vi "MB Open Connection.vi"(11 "Test Object in":T1) -> (0 "error out":errorcluster, 3 "Test Object out":T1)   [LabVIEW 2021]
uses:
  TypeDefs/Tester Object.ctl
  <vilib>/NI/Modbus Library/API/Master/Modbus Master.lvclass
  TypeDefs/UIControlReferences.ctl
  <vilib>/Utility/config.llb/Read Key (String).vi
  <vilib>/Utility/config.llb/Read Key (U32).vi
  <vilib>/NI/Modbus Library/API/Wrapper/Create Serial Master.vi
  <vilib>/NI/Modbus Library/API/Wrapper/Create TCP Master.vi
  <vilib>/regexp/Match Regular Expression.xnode
  <vilib>/NI/Modbus Library/API/Wrapper/API Main.lvlib
  <vilib>/Utility/config.llb/NI_LVConfig.lvlib
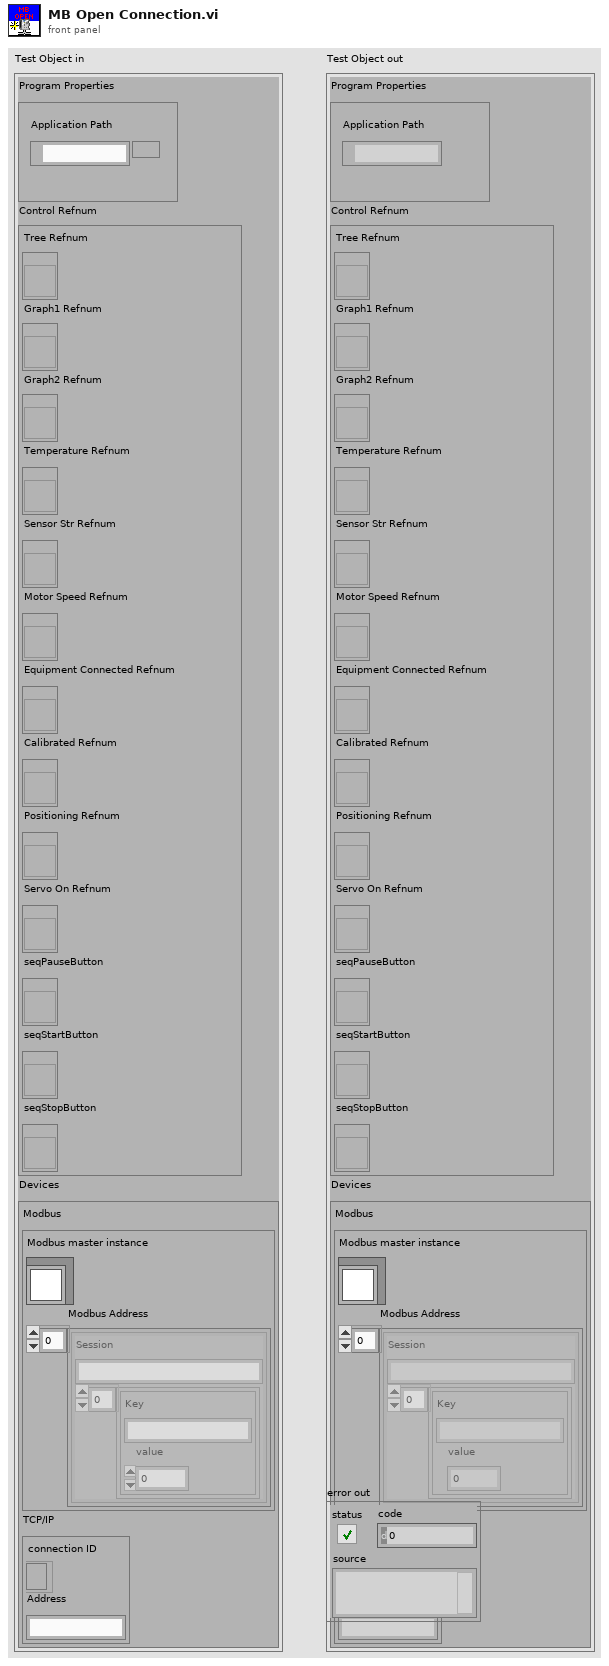
[diagram p1: front panel]
types:
  T1 = typedef "Tester Object.ctl" = cluster{"Program Properties":cluster{"Application Path":path}, "Control Refnum":T2, "Devices":cluster{"Modbus":cluster{"Modbus master instance":refnum<class "Modbus Master.lvclass">, "Modbus Address":cluster{"Session":string, cluster{"Key":string, "value":u32}[]}[]}, "TCP/IP":cluster{"connection ID":refnum<k5>, "Address":string}}}
  T2 = typedef "UIControlReferences.ctl" = cluster{"Tree Refnum ":refnum<vi>, "Graph1 Refnum":refnum<vi>, "Graph2 Refnum":refnum<vi>, "Temperature Refnum":refnum<vi>, "Sensor Str Refnum":refnum<vi>, "Motor Speed Refnum":refnum<vi>, "Equipment Connected Refnum":refnum<vi>, "Calibrated Refnum":refnum<vi>, "Positioning Refnum":refnum<vi>, "Servo On Refnum":refnum<vi>, "seqPauseButton":refnum<vi>, "seqStartButton":refnum<vi>, "seqStopButton":refnum<vi>}
  T3 = typedef "NI_LVConfig.lvlib/Config Data RefNum.ctl" = refnum<k1>
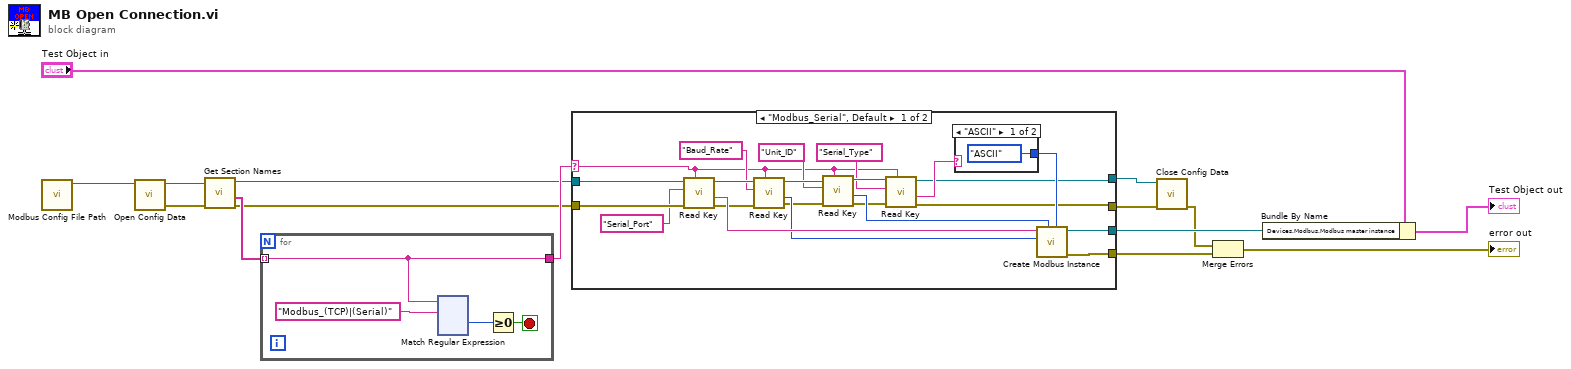
[diagram p0: block diagram]
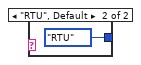
[diagram p2: hidden frame]
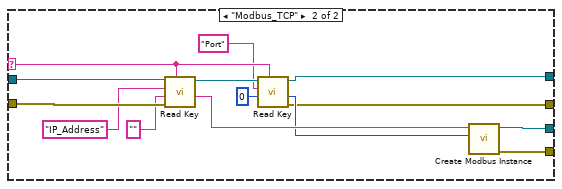
[diagram p3: hidden frame]
diagram:
  n1 = call "Modbus Config File Path.vi"() -> ("appended path out"=w15:path)  [unwired: 11 in]
  n2 = call <vilib>:"Open Config Data.vi"("configuration file path"=w15) -> ("error out"=w13:errorcluster, "refnum"=w14:T3)  [unwired: 8 in, 1 out]
  n3 = call <vilib>:"Get Section Names.vi"("error in (no error)"=w13, "refnum"=w14) -> ("error out"=w9:errorcluster, "section names"=w12:string[], "refnum out"=w10:T3)  [unwired: 7 in]
  n4 = for {
    tunnel: w12 -> [w16] mode=indexing
    tunnel: [w16] -> w11
    stop <- w18 stop-if-true
    n5 = xnode "Match Regular Expression"("input string"=w16, "regular expression"="Modbus_(TCP)|(Serial)") -> ("offset past match"=w17:i32)  [unwired: 4 in, 4 out]
    n6 = Greater Or Equal To 0?(x=w17) -> (x >= 0?=w18:bool)
  }
  n7 = case shown="\"Modbus_Serial\", Default" w11 {
    selector: w11 -> [w141 w167]
    tunnel: w10 -> [w158 w172]
    tunnel: w9 -> [w157 w171]
    tunnel: [w156 w173] -> w6
    tunnel: [w155 w174] -> w5
    tunnel: [w138 w162] -> w4
    tunnel: [w137 w161] -> w3
    frame "Modbus_Serial", Default {
      n8 = call-poly <vilib>:"Read Key.vi"("section"=w141, "error in (no error)"=w157, "key"="Serial_Port", "refnum"=w158) -> ("error out"=w151:errorcluster, "value"=w153:string, "refnum out"=w152:T3)  [unwired: 4 in, 1 out]
      n9 = call-poly <vilib>:"Read Key.vi"("section"=w141, "error in (no error)"=w151, "key"="Baud_Rate", "refnum"=w152) -> ("error out"=w147:errorcluster, "value"=w149:u32, "refnum out"=w148:T3)  [unwired: 4 in, 1 out]
      n10 = call-poly <vilib>:"Read Key.vi"("section"=w141, "error in (no error)"=w147, "key"="Unit_ID", "refnum"=w148) -> ("error out"=w143:errorcluster, "value"=w146:u32, "refnum out"=w144:T3)  [unwired: 4 in, 1 out]
      n11 = call-poly <vilib>:"Read Key.vi"("section"=w141, "error in (no error)"=w143, "key"="Serial_Type", "refnum"=w144) -> ("error out"=w137:errorcluster, "value"=w139:string, "refnum out"=w138:T3)  [unwired: 4 in, 1 out]
      n12 = case shown="\"ASCII\"" w139 {
        tunnel: [enum16{"RTU", "ASCII"}."ASCII" ("serial type") enum16{"RTU", "ASCII"}."RTU" ("serial type")] -> w140
        frame "ASCII" {
        }
        frame "RTU", Default {
        }
      }
      n13 = call-poly <vilib>:"Create Modbus Instance.vi"("serial type"=w140, "unit ID"=w146, "baud rate"=w149, "VISA resource name"=w153) -> ("error out"=w156:errorcluster, "serial master instance"=w155:refnum<class "Modbus Master.lvclass">)  [unwired: 6 in]
    }
    frame "Modbus_TCP" {
      n14 = call-poly <vilib>:"Read Key.vi"("section"=w167, "error in (no error)"=w171, "default value"="", "key"="IP_Address", "refnum"=w172) -> ("value"=w169:string, "refnum out"=w168:T3)  [unwired: 3 in, 2 out]
      n15 = call-poly <vilib>:"Read Key.vi"("section"=w167, "default value"=u32 0, "key"="Port", "refnum"=w168) -> ("error out"=w161:errorcluster, "value"=w166:u32, "refnum out"=w162:T3)  [unwired: 4 in, 1 out]
      n16 = call-poly <vilib>:"Create Modbus Instance.vi"("port (502)"=w166, "address"=w169) -> ("error out"=w173:errorcluster, "TCP master instance"=w174:refnum<class "Modbus Master.lvclass">)  [unwired: 8 in]
    }
  }
  n17 = call <vilib>:"Close Config Data.vi"("error in (no error)"=w3, "refnum"=w4) -> ("error out"=w1:errorcluster)  [unwired: 8 in, 1 out]
  n18 = Merge Errors(w1, w6) -> (→"error out":errorcluster)
  n19 = Bundle By Name(cluster="Test Object in", "Devices.Modbus.Modbus master instance"=w5) -> (→"Test Object out":T1)
